vi "Configure Electrical Calibration Detect.vi"(6 "Module Number (0)":i32, 7 "Enable Auto Detect (F: Disable)":bool, 8 "error in (no error)":errorcluster, 9 "Port (1)":i32=1, 10 "Channel (1)":i32=1, 11 "VISA resource name":refnum<visa-resource-name>) -> (0 "error out":errorcluster, 3 "VISA resource name out":refnum<visa-resource-name>)   [LabVIEW 2020, in "Agilent ENA Series.lvlib"]
doc: "Configures the electrical calibration detect settings.\n\n<B>Note:</B> This VI is only valid for E5061B, E5070B and E5071B."
uses:
  <instrlib>/Agilent ENA Series/Agilent ENA Series.lvlib
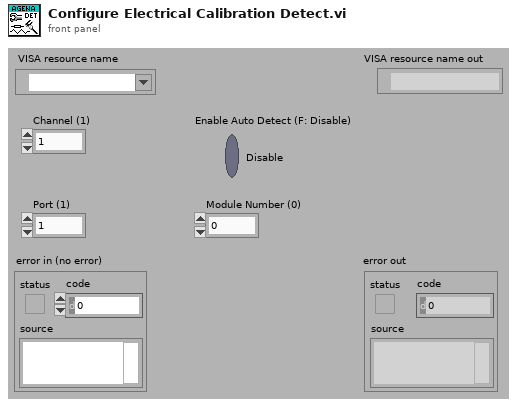
[diagram p1: front panel]
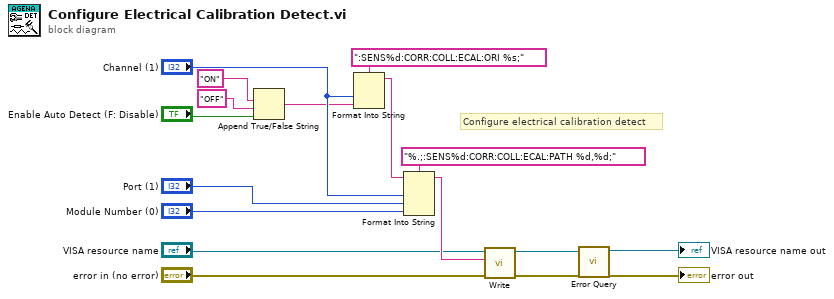
[diagram p0: block diagram]
diagram:
  # "Configure electrical calibration detect"
  n1 = Append True/False String(1:"Enable Auto Detect (F: Disable)", 2:"OFF", 3:"ON") -> (0:w12:string)  [unwired: 1 out]
  n2 = Format Into String(format string=":SENS%d:CORR:COLL:ECAL:ORI %s;", "Channel (1)", w12) -> (resulting string=w11:string)  [unwired: 2 in, 1 out]
  n3 = Format Into String(format string="%.;:SENS%d:CORR:COLL:ECAL:PATH %d,%d;", initial string=w11, "Channel (1)", "Port (1)", "Module Number (0)") -> (resulting string=w5:string)  [unwired: 1 in, 1 out]
  n4 = call <instrlib>:"Write.vi"("error in (no error)"="error in (no error)", "String ()"=w5, "VISA resource name"="VISA resource name") -> ("error out"=w1:errorcluster, "VISA resource name out"=w2:refnum<visa-resource-name>)  [unwired: 6 in, 1 out]
  n5 = call <instrlib>:"Error Query.vi"("error in (no error)"=w1, "VISA resource name"=w2) -> ("error out"=→"error out":errorcluster, "VISA resource name out"=→"VISA resource name out":refnum<visa-resource-name>)  [unwired: 8 out]
